vi "XLP80_Datalog_ContUpdate.vi"(8 "err in":errorcluster) -> (0 "err out":errorcluster)   [LabVIEW 2021]
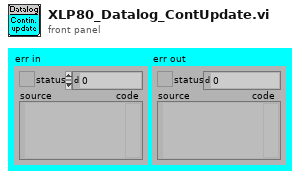
[diagram p1: front panel]
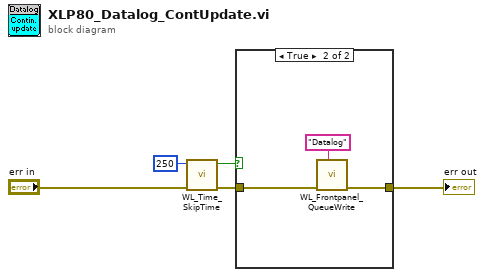
[diagram p0: block diagram]
diagram:
  n1 = call "WL_Time_SkipTime.vi"("err in"="err in", "SkipTime[ms]"=u32 250) -> ("err out"=w3:errorcluster, "Run"=w1:bool)  [unwired: 8 in]
  n2 = case shown="True" w1 {
    tunnel: [w6 w9] -> w4
    tunnel: w3 -> [w6 w8]
    frame False {
    }
    frame True {
      n3 = call "WL_Frontpanel_QueueWrite.vi"("Command (error only)"="Datalog", "err in"=w8) -> ("err out"=w9:errorcluster)  [unwired: 9 in]
    }
  }
  "err out" <- w4
